vi "getCommunicator.vi"(11 "Publisher in":refnum<class "Publisher.lvclass">) -> (2 "Communicator":refnum<class "Communicator.lvclass">, 3 "Publisher out":refnum<class "Publisher.lvclass">)   [LabVIEW 2016, in "Publisher.lvclass"]
uses:
  Publisher.lvclass
  Communicator/Communicator/Communicator.lvclass
  Publisher.lvclass/Publisher.ctl
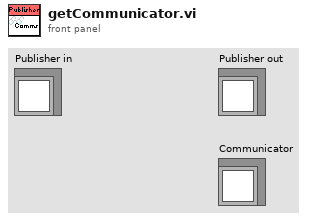
[diagram p1: front panel]
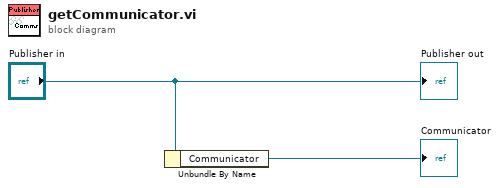
[diagram p0: block diagram]
diagram:
  n1 = Unbundle By Name("Publisher in") -> ("Communicator"=→"Communicator":refnum<class "Communicator.lvclass">)
  "Publisher out" <- "Publisher in"
